vi "R=Base.vi"(8 "Offset":T2, 9 "Matrix":T1 format="%.3f", 11 "Command":string="Reference") -> (0 "error out":errorcluster, 2 "Joints":dbl[](array[numeric])=[0.0, -45.0, 0.0, 45.0, 0.0, 90.0, 0.0], 3 "Matrix":T1 format="%.3f")   [LabVIEW 2013]
uses:
  <vilib>/Analysis/Matrix/Datatypes/RealMatrix.ctl
  ROS/Code/SubVIs/BaxterSide.ctl
  ROS/Code/Console/Servers/ServerSubs/(nist) Arm Globals.vi
  Prim/Fwd Kenimatics - array.vi
  <vilib>/Analysis/Matrix/NI_Matrix.lvlib
panel:
  in  "Ref Point":dbl[](array[numeric])=[0.0, -45.0, 0.0, 90.0, 0.0, 45.0, 0.0]
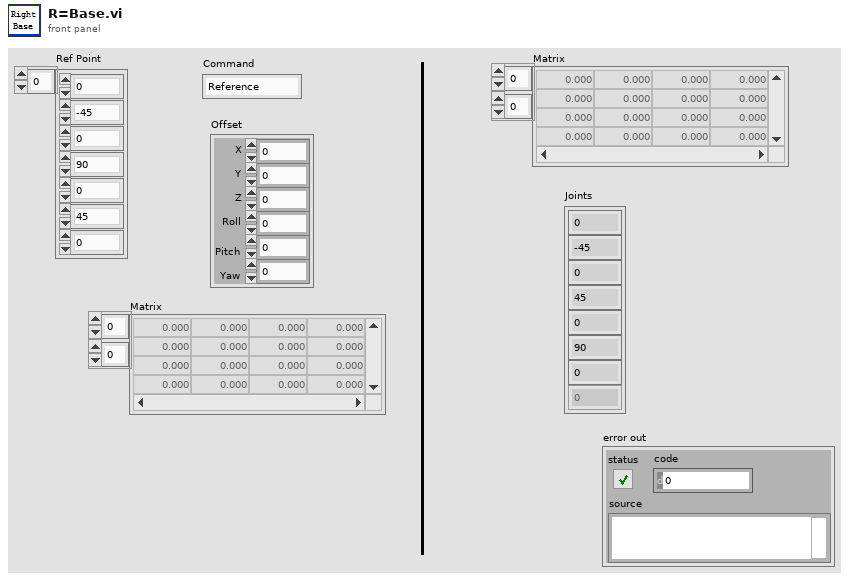
[diagram p1: front panel]
types:
  T1 = typedef "NI_Matrix.lvlib/RealMatrix.ctl" = dbl[][]
  T2 = cluster{"X":dbl, "Y":dbl, "Z":dbl, "Roll":dbl, "Pitch":dbl, "Yaw":dbl}
  T3 = typedef "BaxterSide.ctl" = enum16{"left", "right"}
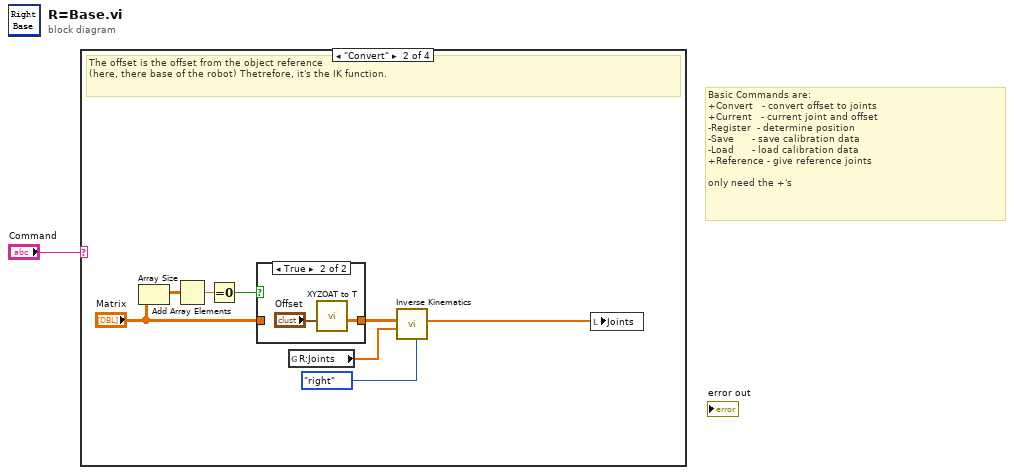
[diagram p0: block diagram]
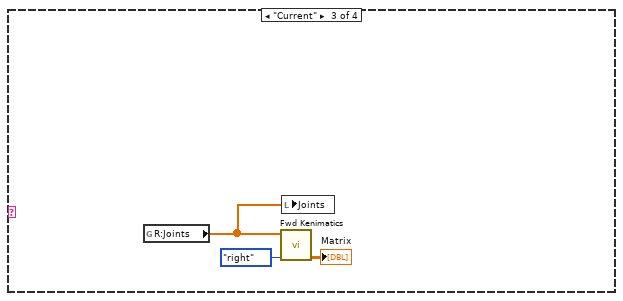
[diagram p4: hidden frame]
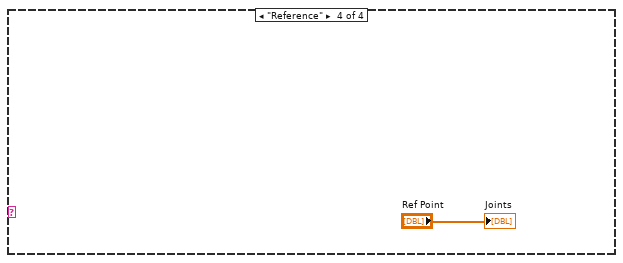
[diagram p5: hidden frame]
diagram:
  # "Basic Commands are:\n+Convert   - convert offset to joints\n+Current   - current joint and offset\n-Register  - determine position\n-Save      - save calibration data\n-Load      - load calibration data\n+Reference - give reference joints\n\nonly need the +'s"
  n1 = case shown="\"Convert\"" "Command" {
    frame Default {
    }
    frame "Convert" {
      # "The offset is the offset from the object reference\n(here, there base of the robot) Thetrefore, it's the IK function."
      n2 = Array Size(array="Matrix") -> ()  [unwired: 1 out]
      n3 = Add Array Elements(numeric array="Matrix") -> (sum=w5:dbl)
      n4 = Equal To 0?(x=w5) -> (x = 0?=w4:bool)
      n5 = case shown="True" w4 {
        tunnel: [w9 w10] -> w6
        tunnel: "Matrix" -> [w9 _]
        frame False {
        }
        frame True {
          n6 = call "XYZOAT to T.vi"("XYZOAT"="Offset") -> ("T"=w10:T1)  [unwired: 10 in]
        }
      }
      n7 = global read "(nist) Arm Globals.vi" "R:Joints"() -> (w2:dbl[])
      n8 = call "Inverse Kinematics.vi"("Side"=BaxterSide."right", "Start"=w2, "Goal-matrix"=w6) -> ("J"=w7:dbl[])  [unwired: 5 in, 3 out]
      n9 = local write "Joints"(w7) -> ()
    }
    frame "Current" {
      n10 = global read "(nist) Arm Globals.vi" "R:Joints"() -> (w12:dbl[])
      n11 = call-poly "Fwd Kenimatics.vi"("Side"=BaxterSide."right", "Joints"=w12) -> ("Matrix"=→"Matrix":T1)  [unwired: 8 in, 1 out]
      n12 = local write "Joints"(w12) -> ()
    }
    frame "Reference" {
      "Joints" <- "Ref Point"
    }
  }
